vi "Log Data.vi"(6 "MinMax_in":dbl[][](array[numeric]), 7 "TriggerTimeStamp":timestamp=timestamp(3569548862.6211414 s since 1904-01-01), 8 "error in (no error)":errorcluster, 9 "Samples to Save In":u32, 10 "Data":waveform(dbl)[](array[waveform]), 11 "Logging Configuration":T1={"Log File Base Path"=path "", "Samples to Save"=0, "Trigger - Threshold"=0.0, "Trigger - Channel"=0, "Always Log"=FALSE, "External Trigger"=FALSE, "External Trigger Armed"=FALSE, "TDMS File Reference"=refnum, "DAQVersion"="", "SWVersion"="", "CircSamples"=0, "BeepWhenComplete"=FALSE, "ChannelConfig"=[], "ActiveChannels"=[], "Title"="", "Description"="", "ChannelNames"=[], "ResponseExtension"=TRUE}) -> (0 "error out":errorcluster, 1 "Samples to Save Out":u32, 4 "MinMax_out":dbl[][](array[numeric]))   [LabVIEW 2017, in "Logging.lvlib"]
doc: "Use the Write To Measurement File Express VI to log data to disk in a LVM file."
uses:
  Logging.lvlib
  Logging Configuration.ctl
  <vilib>/Waveform/WDTOps.llb/WDT Get Waveform Time Array DBL.vi
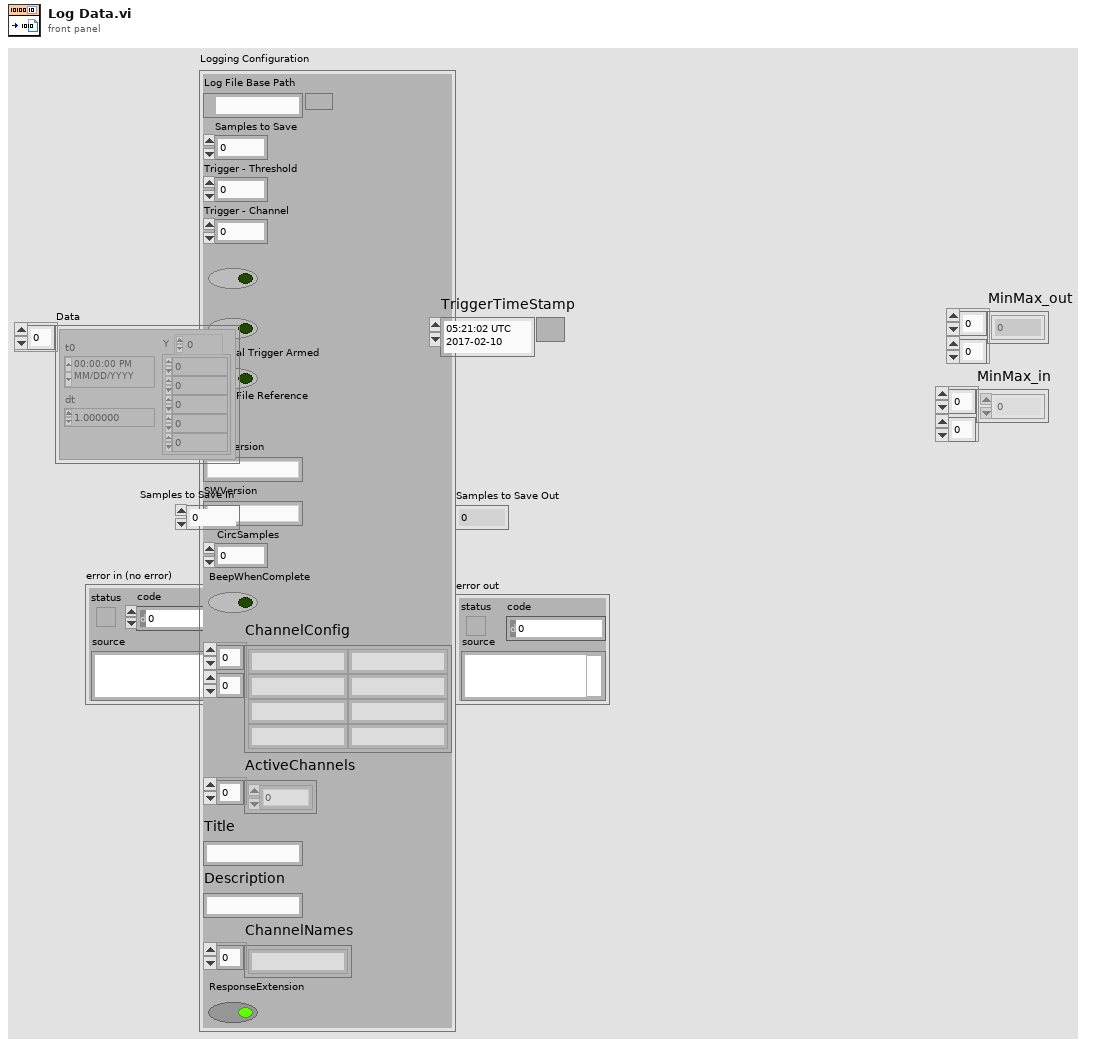
[diagram p1: front panel]
types:
  T1 = typedef "Logging.lvlib/Logging Configuration.ctl" = cluster{"Log File Base Path":path, "Samples to Save":u32, "Trigger - Threshold":dbl, "Trigger - Channel":u32, "Always Log":bool, "External Trigger":bool, "External Trigger Armed":bool, "TDMS File Reference":refnum<k34>, "DAQVersion":string, "SWVersion":string, "CircSamples":u32, "BeepWhenComplete":bool, "ChannelConfig":string[][], "ActiveChannels":i32[], "Title":string, "Description":string, "ChannelNames":string[], "ResponseExtension":bool}
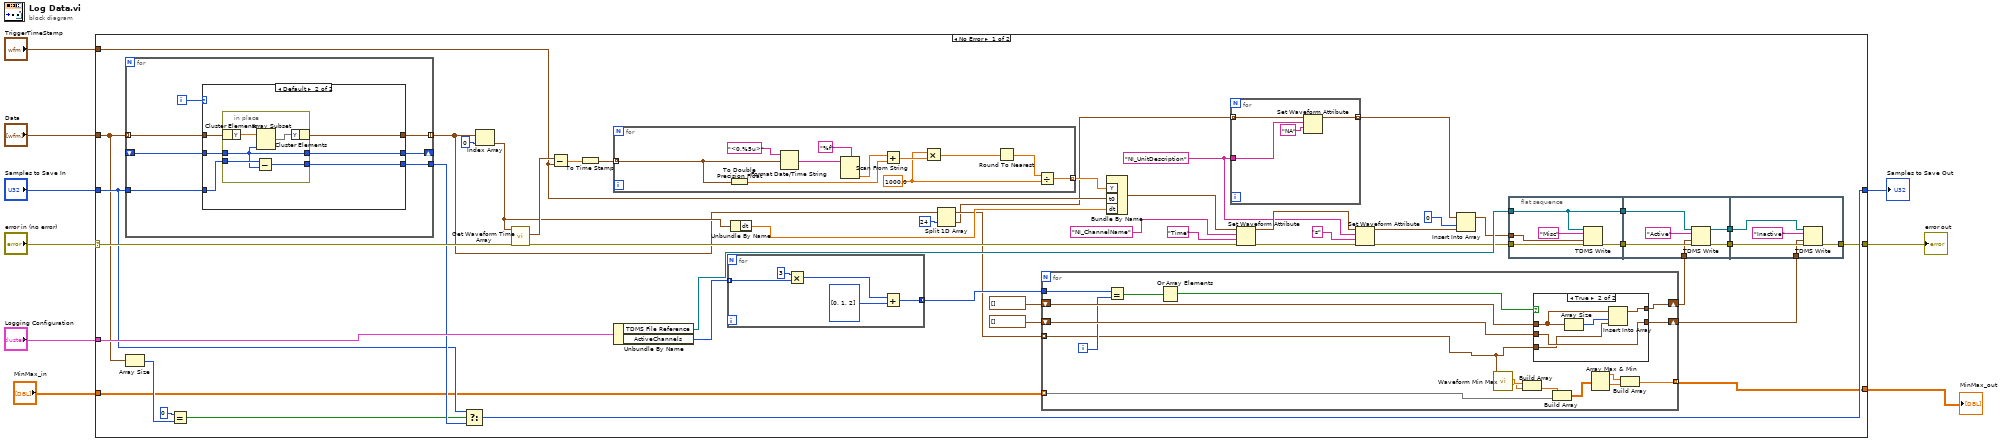
[diagram p0: block diagram]
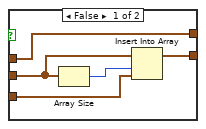
[diagram p2: hidden frame]
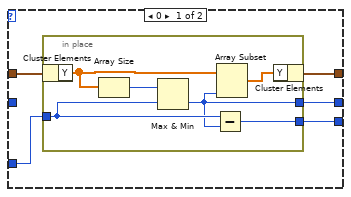
[diagram p3: hidden frame]
diagram:
  n1 = case shown="No Error" "error in (no error)" {
    selector: "error in (no error)" -> [w44 w151]
    tunnel: "Logging Configuration" -> [w57 _]
    tunnel: "Data" -> [w36 _]
    tunnel: "Samples to Save In" -> [w40 w152]
    tunnel: [w42 w152] -> w5
    tunnel: "TriggerTimeStamp" -> [w35 _]
    tunnel: [w33 w151] -> w3
    tunnel: [w11 w150] -> w2
    tunnel: "MinMax_in" -> [w10 w150]
    frame No Error {
      w17 = "NI_UnitDescription" ("name")
      n2 = for {
        tunnel: w36 -> [w126] mode=indexing
        tunnel: w40 -> [w127]
        tunnel: [w125] -> w24 mode=indexing
        tunnel: [w124] -> w41
        shift-right: [w122] -> _
        shift-left: _ -> [w121]
        i -> [w123]
        n3 = case shown="Default" w123 {
          tunnel: w127 -> [w132 w144]
          tunnel: w126 -> [w128 w140]
          tunnel: [w129 w139] -> w125
          tunnel: [w131 w143] -> w124
          tunnel: [w130 w141] -> w122
          tunnel: w121 -> [_ w142]
          frame 0 {
            n4 = in-place {
              in-place-border: w132 -> [w138]
              in-place-border: [w137] -> w131
              in-place-border: [w134] -> w130
              n5 = in-place-cluster #1(w128) -> ("Y"=w136:dbl[])
              n6 = Array Size(array=w136) -> (size(s)=w133:i32)
              n7 = Max & Min(x=w133, y=w138) -> (min(x,y)=w134:u32)  [unwired: 1 out]
              n8 = Subtract(x=w138, y=w134) -> (x-y=w137:u32)
              n9 = Array Subset(array=w136, length=w134) -> (w135:dbl[])  [unwired: 1 in]
              n10 = in-place-cluster #1("Y"=w135) -> (w129:waveform(dbl))
            }
          }
          frame Default {
            n11 = in-place {
              in-place-border: w144 -> [w149]
              in-place-border: [w148] -> w143
              in-place-border: [w145] -> w141
              in-place-border: w142 -> [w145]
              n12 = in-place-cluster #2(w140) -> ("Y"=w147:dbl[])
              n13 = Subtract(x=w149, y=w145) -> (x-y=w148:u32)
              n14 = Array Subset(array=w147, length=w145) -> (w146:dbl[])  [unwired: 1 in]
              n15 = in-place-cluster #2("Y"=w146) -> (w139:waveform(dbl))
            }
          }
        }
      }
      n16 = Array Size(array=w36) -> (size(s)=w38:i32)
      n17 = Equal?(x=0, y=w38) -> (x = y?=w39:bool)
      n18 = Select(t=w40, s=w39, f=w41) -> (s? t:f=w42:u32)
      n19 = Index Array(array=w24, index=0) -> (element=w52:waveform(dbl))
      n20 = call-poly <vilib>:"Get Waveform Time Array.vi"("error in (no error)"=w44, "waveform in"=w52) -> ("error out"=w43:errorcluster, "X array"=w55:timestamp[])  [unwired: 8 in]
      n21 = Subtract(x=w55, y=w35) -> (x-y=w34:dbl[])
      n22 = To Time Stamp(1:w34) -> (0:w54:timestamp[])
      n23 = for {
        tunnel: w54 -> [w119] mode=indexing
        tunnel: [w112] -> w53 mode=indexing
        w111 = 1000.0 ("x")
        n24 = To Double Precision Float(number=w119) -> (double precision float=w115:dbl)
        n25 = Format Date/Time String(time format string (%c)="<0.%5u>", seconds (now)=w119) -> (date/time string=w118:string)  [unwired: 1 in]
        n26 = Scan From String(format string="%f", input string=w118) -> (output 1=w116:dbl)  [unwired: 3 in, 3 out]
        n27 = Add(x=w116, y=w115) -> (x+y=w113:dbl)
        n28 = Multiply(x=w111, y=w113) -> (x*y=w114:dbl)
        n29 = Round To Nearest(number=w114) -> (nearest integer value=w110:dbl)
        n30 = Divide(x=w110, y=w111) -> (x/y=w112:dbl)
      }
      n31 = Unbundle By Name(w57) -> ("TDMS File Reference"=w30:refnum<k34>, "ActiveChannels"=w26:i32[])
      n32 = for {
        tunnel: w26 -> [w66] mode=indexing
        tunnel: [w62] -> w25 mode=concatenating
        n33 = Multiply(x=3, y=w66) -> (x*y=w64:i32)
        n34 = Add(x=w64, y=i32[] [0, 1, 2]) -> (x+y=w62:i32[])
      }
      n35 = Unbundle By Name(w52) -> ("dt"=w45:dbl)
      n36 = Split 1D Array(array=w24, index=24 ("length")) -> (first subarray=w22:waveform(dbl)[], second subarray=w18:waveform(dbl)[])
      n37 = for {
        tunnel: w22 -> [w83] mode=indexing
        tunnel: w25 -> [w99]
        shift-right: [w97] -> w14
        shift-left: waveform(dbl)[] [] -> [w96]
        shift-right: [w94] -> w15
        shift-left: waveform(dbl)[] [] -> [w95]
        tunnel: [w85] -> w11 mode=indexing
        tunnel: w10 -> [w92] mode=indexing
        i -> [w84]
        n38 = Equal?(x=w99, y=w84) -> (x = y?=w98:bool[])
        n39 = Or Array Elements(Boolean array=w98) -> (logical OR=w93:bool)
        n40 = call <vilib>:"Waveform Min Max.vi"("waveform in"=w83) -> ("Y min"=w90:dbl, "Y max"=w91:dbl)  [unwired: 5 in, 4 out]
        n41 = Build Array(w91, w90) -> (w89:dbl[])
        n42 = case shown="True" w93 {
          tunnel: w83 -> [w102 w105]
          tunnel: [w103 w107] -> w97
          tunnel: w96 -> [w103 w106]
          tunnel: w95 -> [w100 w109]
          tunnel: [w104 w109] -> w94
          frame False {
            n43 = Array Size(array=w100) -> (size(s)=w101:i32)
            n44 = Insert Into Array(array=w100, index=w101, new element=w102) -> (w104:waveform(dbl)[])
          }
          frame True {
            n45 = Array Size(array=w106) -> (size(s)=w108:i32)
            n46 = Insert Into Array(array=w106, index=w108, new element=w105) -> (w107:waveform(dbl)[])
          }
        }
        n47 = Build Array(w89, w92) -> (w86:dbl[][])
        n48 = Array Max & Min(array=w86) -> (max value=w88:dbl, min value=w87:dbl)  [unwired: 2 out]
        n49 = Build Array(w88, w87) -> (w85:dbl[])
      }
      n50 = Bundle By Name("Y"=w53, "t0"=w35, "dt"=w45) -> (w51:waveform(dbl))  [unwired: 1 in]
      n51 = for {
        tunnel: w18 -> [w59] mode=indexing
        tunnel: w17 -> [w61]
        tunnel: [w58] -> w16 mode=indexing
        n52 = Set Waveform Attribute(5:"NA" ("name"), 6:w61, 7:w59) -> (3:w58:waveform(dbl))  [unwired: 1 in, 2 out]
      }
      n53 = Set Waveform Attribute(4:w43, 5:"Time" ("name"), 6:"NI_ChannelName" ("name"), 7:w51) -> (0:w46:errorcluster, 3:w48:waveform(dbl))  [unwired: 1 out]
      n54 = Set Waveform Attribute(4:w46, 5:"s" ("name"), 6:w17, 7:w48) -> (0:w28:errorcluster, 3:w20:waveform(dbl))  [unwired: 1 out]
      n55 = Insert Into Array(array=w16, index=0, new element=w20) -> (w19:waveform(dbl)[])
      n56 = flat-sequence {
        tunnel: w30 -> [w71]
        tunnel: w19 -> [w70]
        tunnel: [w71] -> w29
        tunnel: w28 -> [w69]
        tunnel: [w68] -> w27
        tunnel: [w77] -> w32
        tunnel: [w76] -> w31
        tunnel: w29 -> [w75]
        tunnel: w27 -> [w74]
        tunnel: w14 -> [w73]
        tunnel: [w82] -> w33
        tunnel: w32 -> [w81]
        tunnel: w31 -> [w80]
        tunnel: w15 -> [w78]
        frame #0 {
          n57 = TDMS Write(0:w71, 5:"Misc" ("group name in (Untitled)"), 9:w70, 11:w69) -> (15:w68:errorcluster)  [unwired: 2 in, 3 out]
        }
        frame #1 {
          n58 = TDMS Write(0:w75, 5:"Active" ("t"), 9:w73, 11:w74) -> (4:w76:refnum<k34>, 15:w77:errorcluster)  [unwired: 2 in, 2 out]
        }
        frame #2 {
          n59 = TDMS Write(0:w80, 5:"Inactive", 9:w78, 11:w81) -> (15:w82:errorcluster)  [unwired: 2 in, 3 out]
        }
      }
    }
    frame Error {
    }
  }
  "error out" <- w3
  "Samples to Save Out" <- w5
  "MinMax_out" <- w2
